vi "room path sel.vi"(10 "room name":string) -> (1 "go next":T1, 2 "go room path":T1, 4 "recy dir":bool, 6 "block dir":bool)   [LabVIEW 2019]
uses:
  ctl/path name.ctl
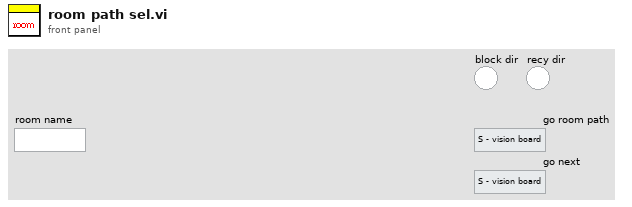
[diagram p1: front panel]
types:
  T1 = typedef "path name.ctl" = enum16{"S - vision board", "vision board - s out", "s out - room center", "room center - R1", "room center - R2", "room center - R3", "room center - R4", "room center - R5", "R1 - room center", "R2 - room center", "R3 - room center", "R4 - room center", "R5 - room center", "room center - S out", "S-out - recycle", "recycle - S-out", "S-out - s", "s - s-out", "board - box", "box - board", "S out - board", "R1 - R1 d", "R5d - R5", "R3.4-R3", "R3 - R3.2", "- align", "- align.5", "R2 - R2.d", "center align"}
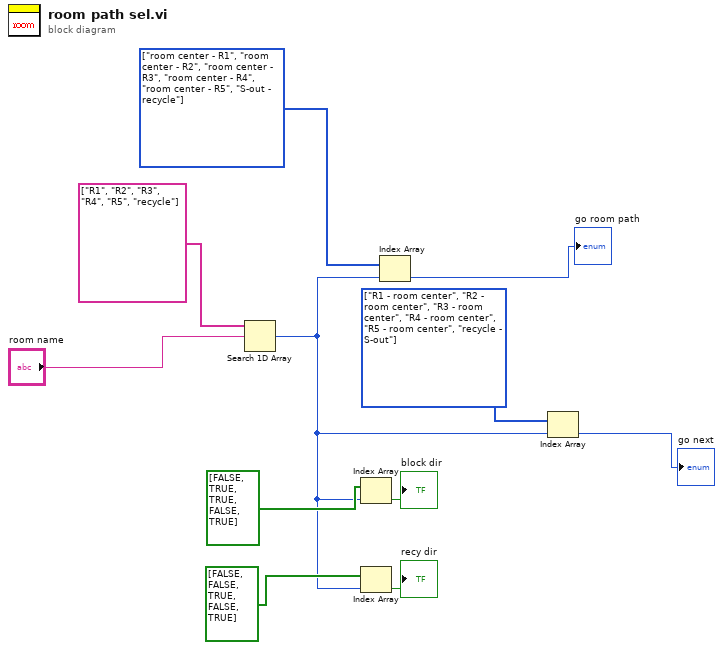
[diagram p0: block diagram]
diagram:
  w6 = T1[] [enum."R1 - room center", enum."R2 - room center", enum."R3 - room center", enum."R4 - room center", enum."R5 - room center", enum."recycle - S-out"] items=["S - vision board", "vision board - s out", "s out - room center", "room center - R1", "room center - R2", "room center - R3", "room center - R4", "room center - R5", "R1 - room center", "R2 - room center", "R3 - room center", "R4 - room center", "R5 - room center", "room center - S out", "S-out - recycle", "recycle - S-out", "S-out - s", "s - s-out", "board - box", "box - board", "S out - board", "R1 - R1 d", "R5d - R5", "R3.4-R3", "R3 - R3.2", "- align", "- align.5", "R2 - R2.d", "center align"] ("Array")
  w9 = T1[] [enum."room center - R1", enum."room center - R2", enum."room center - R3", enum."room center - R4", enum."room center - R5", enum."S-out - recycle"] items=["S - vision board", "vision board - s out", "s out - room center", "room center - R1", "room center - R2", "room center - R3", "room center - R4", "room center - R5", "R1 - room center", "R2 - room center", "R3 - room center", "R4 - room center", "R5 - room center", "room center - S out", "S-out - recycle", "recycle - S-out", "S-out - s", "s - s-out", "board - box", "box - board", "S out - board", "R1 - R1 d", "R5d - R5", "R3.4-R3", "R3 - R3.2", "- align", "- align.5", "R2 - R2.d", "center align"] ("Array")
  n1 = Search 1D Array(1D array=string[] ["R1", "R2", "R3", "R4", "R5", "recycle"], element="room name") -> (index of element=w3:i32)  [unwired: 1 in]
  n2 = Index Array(array=bool[] [FALSE, TRUE, TRUE, FALSE, TRUE], index=w3) -> (element=→"block dir":bool)
  n3 = Index Array(array=bool[] [FALSE, FALSE, TRUE, FALSE, TRUE], index=w3) -> (element=→"recy dir":bool)
  n4 = Index Array(array=w9, index=w3) -> (element=→"go room path":T1)
  n5 = Index Array(array=w6, index=w3) -> (element=→"go next":T1)
